vi "Generate Picoscope 2000a Series Data.vi"(0 "handle in":i16, 1 "Max ADC":i16=32767, 2 "Ch1 Range Index":u16, 3 "Ch2 Range Index":u16, 4 "Actual Sample Interval":dbl, 5 "error in (no error)":errorcluster, 6 "t0":timestamp, 8 "Channel 1 Buff In":refnum<data-value>, 10 "Channel 2 Buff In":refnum<data-value>) -> (7 "next t0":timestamp, 9 "Channel 1 Buff Out":refnum<data-value>, 11 "Channel 2 Buff Out":refnum<data-value>, 14 "handle out":i16, 16 "Graph Data":waveform(dbl)[](array[waveform]), 19 "error out":errorcluster)   [LabVIEW 2016, in "Acquisition.lvlib"]
doc: "Generates sample waveforms according to the signal type in the HW Config input."
uses:
  Acquisition.lvlib
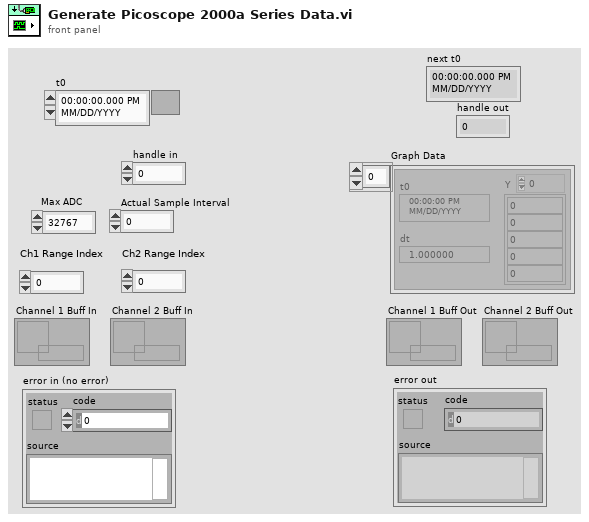
[diagram p1: front panel]
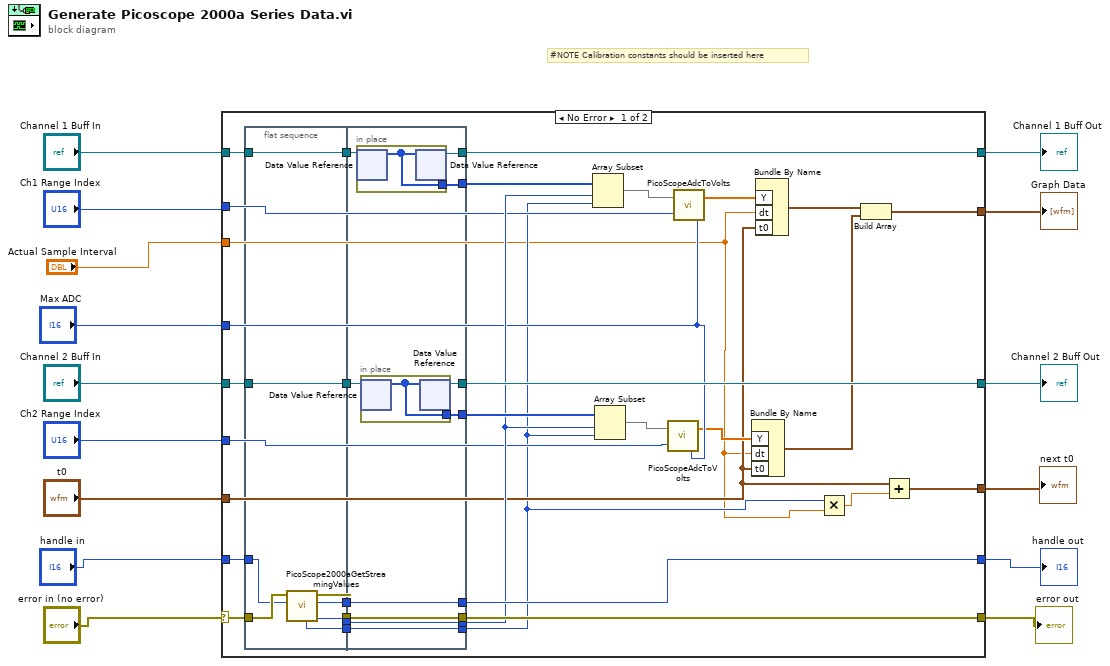
[diagram p0: block diagram]
diagram:
  # "#NOTE Calibration constants should be inserted here"
  n1 = case shown="No Error" "error in (no error)" {
    selector: "error in (no error)" -> [w39 w71]
    tunnel: [w40 w71] -> w14
    tunnel: [w47 _] -> w7
    tunnel: "Channel 1 Buff In" -> [w46 w68]
    tunnel: [w45 w68] -> w12
    tunnel: "handle in" -> [w38 w70]
    tunnel: [w37 w70] -> w10
    tunnel: "Channel 2 Buff In" -> [w44 w69]
    tunnel: [w42 w69] -> w8
    tunnel: "Actual Sample Interval" -> [w22 _]
    tunnel: "Ch1 Range Index" -> [w32 _]
    tunnel: "Max ADC" -> [w33 _]
    tunnel: "Ch2 Range Index" -> [w29 _]
    tunnel: "t0" -> [w26 _]
    tunnel: [w23 _] -> w1
    frame No Error {
      n2 = flat-sequence {
        tunnel: w46 -> [w49]
        tunnel: w44 -> [w48]
        tunnel: w39 -> [w54]
        tunnel: w38 -> [w53]
        tunnel: [w49] -> w21
        tunnel: [w48] -> w20
        tunnel: [w55] -> w19
        tunnel: [w52] -> w18
        tunnel: [w51] -> w17
        tunnel: [w50] -> w16
        tunnel: [w62] -> w24
        tunnel: [w63] -> w36
        tunnel: [w64] -> w37
        tunnel: [w65] -> w40
        tunnel: [w56] -> w41
        tunnel: [w57] -> w42
        tunnel: [w61] -> w43
        tunnel: [w60] -> w45
        tunnel: w21 -> [w59]
        tunnel: w20 -> [w58]
        tunnel: w19 -> [w65]
        tunnel: w18 -> [w64]
        tunnel: w17 -> [w63]
        tunnel: w16 -> [w62]
        frame #0 {
          n3 = call "PicoScope2000aGetStreamingValues.vi"("handle in"=w53, "error in"=w54) -> ("Start Index"=w51:u32, "handle out"=w52:i16, "error out"=w55:errorcluster, "Number of Samples"=w50:i32)  [unwired: 4 in, 2 out]
        }
        frame #1 {
          n4 = in-place {
            in-place-border: [w67] -> w61
            n5 = in-place-dvr #1(w59) -> (w67:i16[])  [unwired: 1 out]
            n6 = in-place-dvr #1(w67) -> (w60:refnum<data-value>)  [unwired: 1 out]
          }
          n7 = in-place {
            in-place-border: [w66] -> w56
            n8 = in-place-dvr #2(w58) -> (w66:i16[])  [unwired: 1 out]
            n9 = in-place-dvr #2(w66) -> (w57:refnum<data-value>)  [unwired: 1 out]
          }
        }
      }
      n10 = Array Subset(array=w43, index=w36, length=w24) -> (w35:i16[])
      n11 = Array Subset(array=w41, index=w36, length=w24) -> (w31:i16[])
      n12 = call "PicoScopeAdcToVolts.vi"("Max ADC"=w33, "Range Index"=w29, "Data"=w31) -> ("Data (Volts)"=w30:dbl[])
      n13 = call "PicoScopeAdcToVolts.vi"("Max ADC"=w33, "Range Index"=w32, "Data"=w35) -> ("Data (Volts)"=w34:dbl[])
      n14 = Bundle By Name("Y"=w30, "dt"=w22, "t0"=w26) -> (w27:waveform(dbl))  [unwired: 1 in]
      n15 = Bundle By Name("Y"=w34, "dt"=w22, "t0"=w26) -> (w28:waveform(dbl))  [unwired: 1 in]
      n16 = Multiply(x=w24, y=w22) -> (x*y=w25:dbl)
      n17 = Build Array(w28, w27) -> (w47:waveform(dbl)[])
      n18 = Add(x=w26, y=w25) -> (x+y=w23:timestamp)
    }
    frame Error {
    }
  }
  "error out" <- w14
  "Graph Data" <- w7
  "Channel 1 Buff Out" <- w12
  "handle out" <- w10
  "Channel 2 Buff Out" <- w8
  "next t0" <- w1
